vi "NEW_Set Steer Motors.vi"(5 "Disable":bool, 6 "PPR":dbl=1024.0, 8 "Steer Control Mode":T3, 9 "Specific Module Data":T1[](array[typedef])=[{"Motor Pos"=enum."Left-Front", "CAN Bus"="", "Drive ID"=5, "Azimuth ID"=1, "CanCoder ID"=1, "CanCoder Offset"=283.711}, {"Motor Pos"=enum."Right-Front", "CAN Bus"="", "Drive ID"=6, "Azimuth ID"=2, "CanCoder ID"=2, "CanCoder Offset"=79.695}, {"Motor Pos"=enum."Right-Back", "CAN Bus"="", "Drive ID"=7, "Azimuth ID"=3, "CanCoder ID"=3, "CanCoder Offset"=319.746}, {"Motor Pos"=enum."Left-Back", "CAN Bus"="", "Drive ID"=7, "Azimuth ID"=3, "CanCoder ID"=3, "CanCoder Offset"=319.746}], 10 "Swerve Data":T9 {"Back Right"."Angle" scale format="%.3f"; "Back Right"."Velocity" scale=-1.0..1.0 scale format="%.1f"; "Back Left"."Angle" scale format="%.3f"; "Back Left"."Velocity" scale=-1.0..1.0 scale format="%.1f"; "Front Left"."Angle" scale format="%.3f"; "Front Left"."Velocity" scale=-1.0..1.0 scale format="%.1f"; "Front Right"."Angle" scale format="%.3f"; "Front Right"."Velocity" scale=-1.0..1.0 scale format="%.1f"}, 11 "Steer Refs":T4[](array[typedef])) -> (1 "Encoder Counts Out":dbl[](array[numeric]), 3 "Array Out":T4[](array[typedef]))   [LabVIEW 2020, in "SwerveDrive_ACT.lvlib"]
uses:
  SwerveDrive_ACT.lvlib
  Shared Code/TypeDefs/Cluster_Swerve 4 Steer and Velocity.ctl
  Shared Code/TypeDefs/Cluster_Module Velocity-Direction-Rotations.ctl
  Shared Code/TypeDefs/Level_Velocity plus-minus 1.ctl
  Shared Code/TypeDefs/Dial_Compase heading unit circle CCW positive.ctl
  <vilib>/Rock Robotics/WPI/MotorControl/WPI_MotorControlDeviceRef.ctl
  <vilib>/Rock Robotics/WPI/MotorControl/WPI_MotorControlType.ctl
  <vilib>/Rock Robotics/SystemInterfaces/DIO/FPGA_DIOPWMChannel.ctl
  <vilib>/Rock Robotics/WPI/PWM/WPI_PWMDeadband.ctl
  <vilib>/Rock Robotics/SystemInterfaces/DIO/FPGA_DIOChannel.ctl
  Type Defs/ENUM_Steer Mode Select.ctl
  Shared Code/TypeDefs/Cluster_Module Specific Config Data.ctl
  Shared Code/TypeDefs/ENUM_Motor Index.ctl
  <vilib>/Rock Robotics/WPI/ThirdParty/Phoenix-LabVIEW/Motor Controller/Controls/CTRE_Phoenix_MotorControl_ControlMode.ctl
panel:
  # "\"Front\" of Robot"
  # "Right Hand Rule"
  # "X"
  # "+CCW"
  # "Y"
  # "(0,0)"
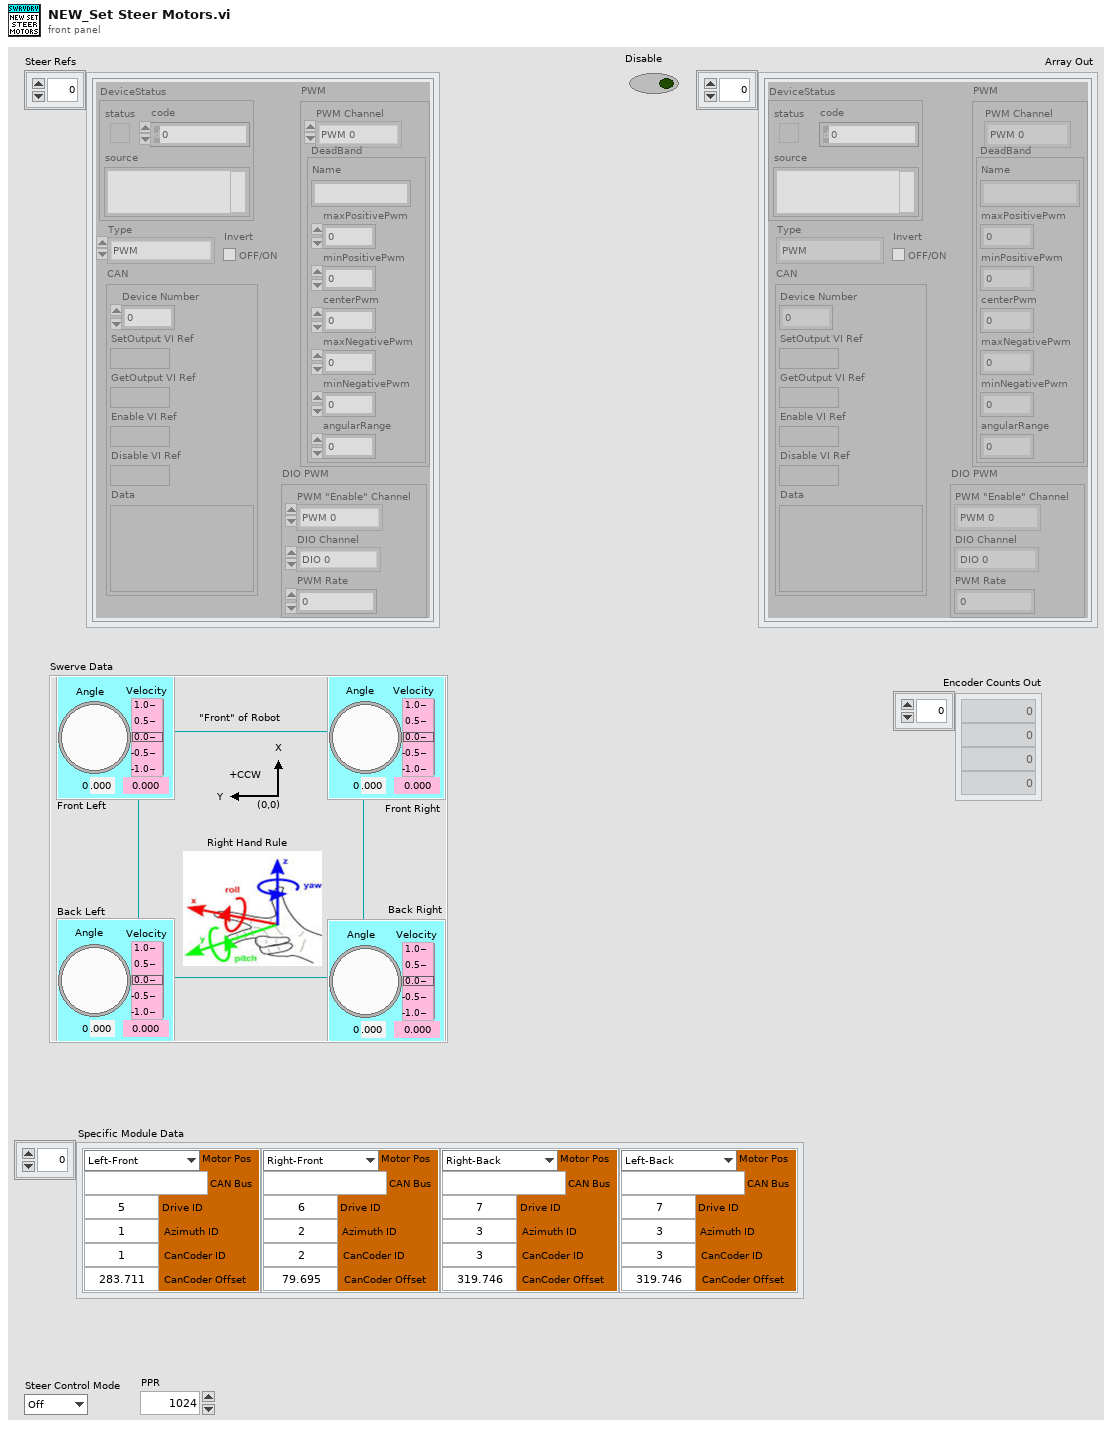
[diagram p1: front panel]
types:
  T1 = typedef "Cluster_Module Specific Config Data.ctl" = cluster{"Motor Pos":T2, "CAN Bus":string, "Drive ID":u8, "Azimuth ID":u8, "CanCoder ID":u8, "CanCoder Offset":dbl}
  T2 = typedef "ENUM_Motor Index.ctl" = enum16{"Left-Front", "Right-Front", "Left-Back", "Right-Back"}
  T3 = typedef "ENUM_Steer Mode Select.ctl" = enum16{"Off", "Hold", "Steer"}
  T4 = typedef "WPI_MotorControlDeviceRef.ctl" = cluster{"DeviceStatus":errorcluster, "Type":T5, "PWM":cluster{"PWM Channel":T6, "DeadBand":T7}, "CAN":cluster{"Device Number":u8, "SetOutput VI Ref":variant, "GetOutput VI Ref":variant, "Enable VI Ref":variant, "Disable VI Ref":variant, "Data":variant}, "Invert":bool, "DIO PWM":cluster{"PWM \"Enable\" Channel":T6, "DIOChannel":T8, "PWM Rate":dbl}}
  T5 = typedef "WPI_MotorControlType.ctl" = enum16{"PWM", "CAN", "DIO PWM"}
  T6 = typedef "FPGA_DIOPWMChannel.ctl" = enum8{"PWM 0", "PWM 1", "PWM 2", "PWM 3", "PWM 4", "PWM 5", "PWM 6", "PWM 7", "PWM 8", "PWM 9", "PWM MXP 0", "PWM MXP 1", "PWM MXP 2", "PWM MXP 3", "PWM MXP 4", "PWM MXP 5", "PWM MXP 6", "PWM MXP 7", "PWM MXP 8", "PWM MXP 9", "Invalid"}
  T7 = typedef "WPI_PWMDeadband.ctl" = cluster{"Name":string, "maxPositivePwm":i32, "minPositivePwm":i32, "centerPwm":i32, "maxNegativePwm":i32, "minNegativePwm":i32, "angularRange":u16}
  T8 = typedef "FPGA_DIOChannel.ctl" = enum8{"DIO 0", "DIO 1", "DIO 2", "DIO 3", "DIO 4", "DIO 5", "DIO 6", "DIO 7", "DIO 8", "DIO 9", "DIO MXP 0", "DIO MXP 1", "DIO MXP 2", "DIO MXP 3", "DIO MXP 4", "DIO MXP 5", "DIO MXP 6", "DIO MXP 7", "DIO MXP 8", "DIO MXP 9", "DIO MXP 10", "DIO MXP 11", "DIO MXP 12", "DIO MXP 13", "DIO MXP 14", "DIO MXP 15", "SPI Port CS1", "SPI Port CS2", "SPI Port CS3", "SPI Port MISO", "SPI Port MOSI", "Invalid"}
  T9 = typedef "Cluster_Swerve 4 Steer and Velocity.ctl" = cluster{"Front Right":T10, "Front Left":T10, "Back Left":T10, "Back Right":T10}
  T10 = typedef "Cluster_Module Velocity-Direction-Rotations.ctl" = cluster{"Velocity":T11, "Angle":T12, "Rotations Count":dbl}
  T11 = typedef "Level_Velocity plus-minus 1.ctl" = dbl
  T12 = typedef "Dial_Compase heading unit circle CCW positive.ctl" = dbl
  T13 = typedef "CTRE_Phoenix_MotorControl_ControlMode.ctl" = u16
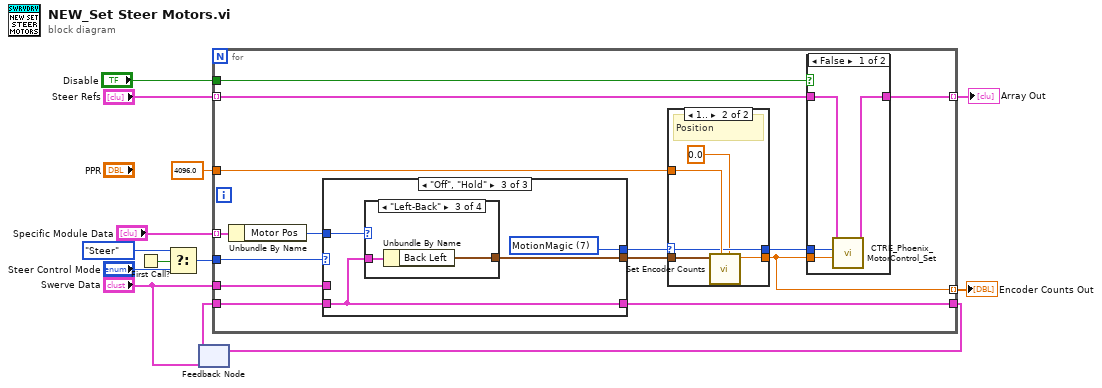
[diagram p0: block diagram]
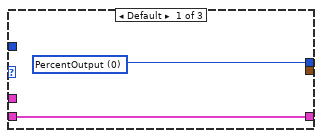
[diagram p3: hidden frame]
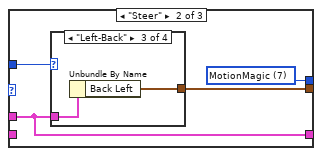
[diagram p4: hidden frame]
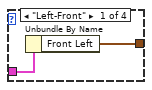
[diagram p5: hidden frame]
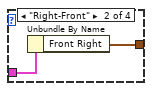
[diagram p6: hidden frame]
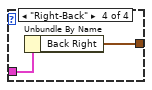
[diagram p7: hidden frame]
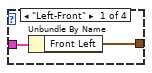
[diagram p8: hidden frame]
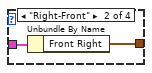
[diagram p9: hidden frame]
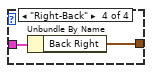
[diagram p10: hidden frame]
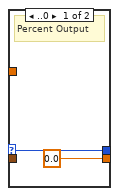
[diagram p11: hidden frame]
diagram:
  n1 = First Call?() -> (First Call?: T/F=w10:bool)
  n2 = Select(t=ENUM_Steer_Mode_Select."Steer" ("Steer Control Mode"), s=w10, f="Steer Control Mode") -> (s? t:f=w7:T3)
  n3 = feedback #1("Swerve Data") -> (w11:T9)
  n4 = for {
    tunnel: "Steer Refs" -> [w27] mode=indexing
    tunnel: "Swerve Data" -> [w24]
    tunnel: [w26] -> w13 mode=indexing
    tunnel: w7 -> [w25]
    tunnel: 4096.0 ("PPR") -> [w22]
    tunnel: "Specific Module Data" -> [w23] mode=indexing
    tunnel: w11 -> [w20]
    tunnel: [w19] -> w5
    tunnel: [w16] -> w4 mode=indexing
    tunnel: "Disable" -> [w15]
    n5 = Unbundle By Name(w23) -> ("Motor Pos"=w14:T2)
    n6 = case shown="\"Off\", \"Hold\"" w25 {
      tunnel: [w34 w38 w50] -> w18
      tunnel: w24 -> [_ w35 _]
      tunnel: w14 -> [_ w37 w49]
      tunnel: [_ w36 w48] -> w21
      tunnel: w20 -> [w33 _ w47]
      tunnel: [w33 w35 w47] -> w19
      frame Default {
        w34 = T13 0 items=["PercentOutput"=0, "Position"=1, "Velocity"=2, "Current"=3, "Follower"=5, "MotionProfile"=6, "MotionMagic"=7, "MotionProfileArc"=10, "Disabled"=15] ("Control Mode")
      }
      frame "Steer" {
        w38 = T13 7 items=["PercentOutput"=0, "Position"=1, "Velocity"=2, "Current"=3, "Follower"=5, "MotionProfile"=6, "MotionMagic"=7, "MotionProfileArc"=10, "Disabled"=15] ("Control Mode")
        n7 = case shown="\"Left-Back\"" w37 {
          tunnel: w35 -> [w40 w42 w44 w46]
          tunnel: [w39 w41 w43 w45] -> w36
          frame "Left-Front" {
            n8 = Unbundle By Name(w40) -> ("Front Left"=w39:T10)
          }
          frame "Right-Front" {
            n9 = Unbundle By Name(w42) -> ("Front Right"=w41:T10)
          }
          frame "Left-Back" {
            n10 = Unbundle By Name(w44) -> ("Back Left"=w43:T10)
          }
          frame "Right-Back" {
            n11 = Unbundle By Name(w46) -> ("Back Right"=w45:T10)
          }
        }
      }
      frame "Off", "Hold" {
        w50 = T13 7 items=["PercentOutput"=0, "Position"=1, "Velocity"=2, "Current"=3, "Follower"=5, "MotionProfile"=6, "MotionMagic"=7, "MotionProfileArc"=10, "Disabled"=15] ("Control Mode")
        n12 = case shown="\"Left-Back\"" w49 {
          tunnel: w47 -> [w52 w54 w56 w58]
          tunnel: [w51 w53 w55 w57] -> w48
          frame "Left-Front" {
            n13 = Unbundle By Name(w52) -> ("Front Left"=w51:T10)
          }
          frame "Right-Front" {
            n14 = Unbundle By Name(w54) -> ("Front Right"=w53:T10)
          }
          frame "Left-Back" {
            n15 = Unbundle By Name(w56) -> ("Back Left"=w55:T10)
          }
          frame "Right-Back" {
            n16 = Unbundle By Name(w58) -> ("Back Right"=w57:T10)
          }
        }
      }
    }
    n17 = case shown="1.." w18 {
      selector: w18 -> [w59 w62]
      tunnel: w21 -> [_ w64]
      tunnel: w22 -> [_ w63]
      tunnel: [0.0 ("Encder Count Set") w65] -> w16
      tunnel: [w59 w62] -> w17
      frame ..0 {
        # "Percent Output"
      }
      frame 1.. {
        # "Position"
        n18 = call "Set Encoder Counts.vi"("Encoder Count at Zero"=0.0, "PPR"=w63, "Angle(0-1) in"=w64) -> ("Encder Count Set"=w65:dbl)  [unwired: 8 in]
      }
    }
    n19 = case shown="False" w15 {
      tunnel: w27 -> [w31 w32]
      tunnel: [w30 w32] -> w26
      tunnel: w17 -> [w29 _]
      tunnel: w16 -> [w28 _]
      frame False {
        n20 = call <vilib>:"CTRE_Phoenix_MotorControl_Set.vi"("Output"=w28, "Control Mode"=w29, "PhoenixMotorControlDevRef"=w31) -> ("PhoenixMotorControlDevRef"=w30:T4)  [unwired: 7 in, 1 out]
      }
      frame True {
      }
    }
  }
  "Array Out" <- w13
  "Encoder Counts Out" <- w4
  n21 = feedback-in #1(w5) -> ()
